vi "Instr_InitObject.vi"(8 "error in (no error)":errorcluster, 9 "Instrument Configuration":variant, 10 "Instrument address":refnum<visa-resource-name>, 11 "KE3700A in":refnum<class "KE3706A.lvclass">) -> (0 "error out":errorcluster, 3 "KE3700A out":refnum<class "KE3706A.lvclass">)   [LabVIEW 2013, in "KE3706A.lvclass"]
uses:
  KE3706A.lvclass
  Switching.lvclass
  InstrumentSetup.vi
  KE3706A_CommandsGlobal.vi
  InstrControl.lvclass
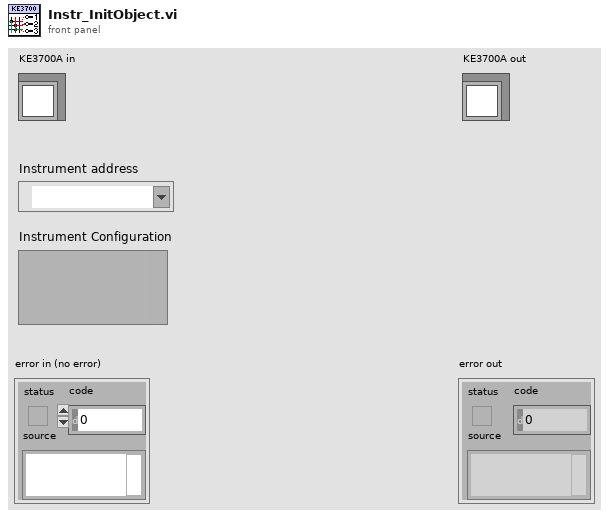
[diagram p1: front panel]
types:
  T1 = cluster{"Mux1 slot":string, "Mux2 slot":string, "KE3706A":refnum<class "KE3706A.lvclass">}
  T2 = cluster{"Instrument name":string, "Instrument type":u16, "Command \"Matrix Reset\"":string, "Command \"connect channel exclusively\"":string, "Command \"Disconnect all MUX Channels\"":string, "Mux1 slot":string, "Mux2 slot":string}
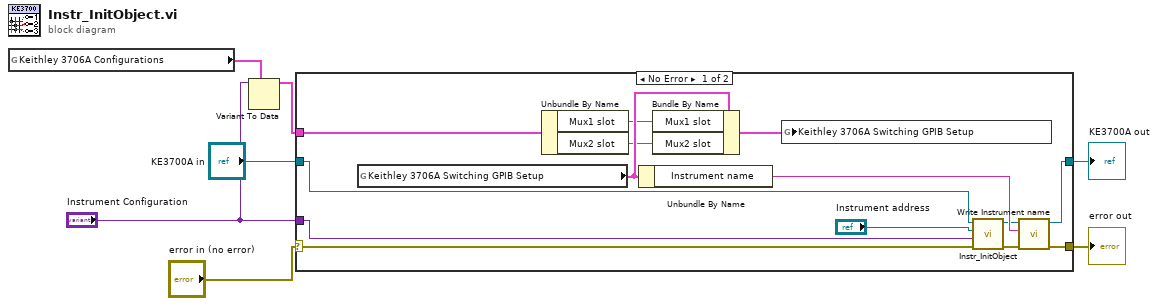
[diagram p0: block diagram]
diagram:
  n1 = global read "InstrumentSetup.vi" "Keithley 3706A Configurations"() -> (w3:T1)
  n2 = Variant To Data(type=w3, Variant="Instrument Configuration") -> (data=w2:T1)  [unwired: 1 in, 1 out]
  n3 = case shown="No Error" "error in (no error)" {
    selector: "error in (no error)" -> [w9 w23]
    tunnel: "KE3700A in" -> [w8 w22]
    tunnel: [w12 w23] -> w5
    tunnel: [w13 w22] -> w4
    tunnel: w2 -> [w16 _]
    tunnel: "Instrument Configuration" -> [w10 _]
    frame No Error {
      n4 = global read "KE3706A_CommandsGlobal.vi" "Keithley 3706A Switching GPIB Setup"() -> (w20:T2)
      n5 = Unbundle By Name(w16) -> ("Mux1 slot"=w19:string, "Mux2 slot"=w18:string)
      n6 = Unbundle By Name(w20) -> ("Instrument name"=w21:string)
      n7 = Bundle By Name(cluster=w20, "Mux1 slot"=w19, "Mux2 slot"=w18) -> (w17:T2)
      n8 = global write "KE3706A_CommandsGlobal.vi" "Keithley 3706A Switching GPIB Setup"(w17) -> ()
      n9 = call-parent "Instr_InitObject.vi"("error in (no error)"=w9, "Instrument Configuration"=w10, "Instrument address"="Instrument address", "Switching in"=w8) -> ("error out"=w14:errorcluster, "Switching out"=w15:refnum<class "KE3706A.lvclass">)  [unwired: 6 in]
      n10 = call-dynamic "Write Instrument name.vi"("error in (no error)"=w14, "Instrument name"=w21, "InstControl in"=w15) -> ("error out"=w12:errorcluster, "InstControl out"=w13:refnum<class "KE3706A.lvclass">)  [unwired: 7 in]
    }
    frame Error {
    }
  }
  "error out" <- w5
  "KE3700A out" <- w4
